vi "AH2500_Check_Queue.vi"(7 "error in (no error)":errorcluster caption="Fehler (Eingang, kein Fehler)", 10 "Queue":refnum<queue> caption="5T Queue") -> (0 "error out":errorcluster caption="Fehler (Ausgang)", 1 "AH2500-Control":T1, 3 "New Entries?":bool)   [LabVIEW 2019]
uses:
  AH2500/AH2500-Control.ctl
panel:
  out "Numerisch":i32
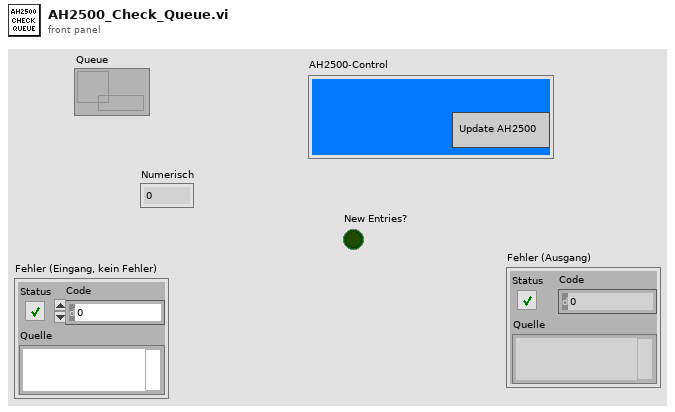
[diagram p1: front panel]
types:
  T1 = typedef "AH2500-Control.ctl" = cluster{"Update AH2500":bool}
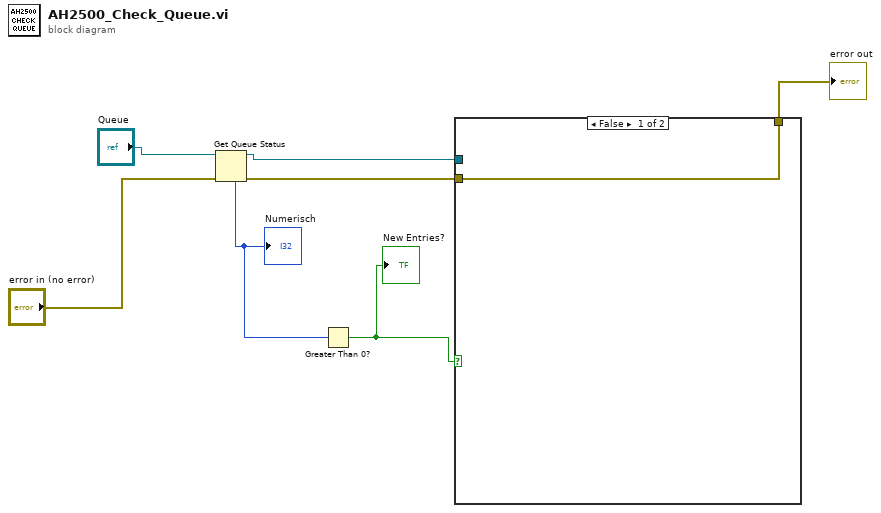
[diagram p0: block diagram]
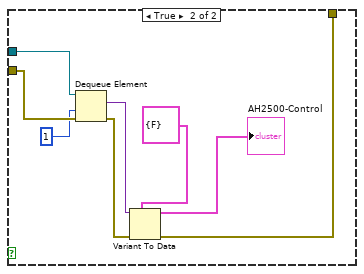
[diagram p2: hidden frame]
diagram:
  n1 = Get Queue Status(queue="Queue", error in (no error)="error in (no error)") -> (queue out=w6:refnum<queue>, error out=w5:errorcluster, # elements in queue=w3:i32)  [unwired: 1 in, 5 out]
  "Numerisch" <- w3
  n2 = Greater Than 0?(x=w3) -> (x > 0?=w2:bool)
  "New Entries?" <- w2
  n3 = case shown="False" w2 {
    tunnel: w6 -> [_ w15]
    tunnel: w5 -> [w8 w16]
    tunnel: [w8 w9] -> w1
    frame False {
    }
    frame True {
      n4 = Dequeue Element(queue=w15, timeout in ms (-1)=1, error in (no error)=w16) -> (element=w13:variant, error out=w12:errorcluster)  [unwired: 2 out]
      n5 = Variant To Data(error in=w12, type=T1 {"Update AH2500"=FALSE} ("AH2500-Control"), Variant=w13) -> (data=→"AH2500-Control":T1, error out=w9:errorcluster)
    }
  }
  "error out" <- w1
